vi "Arduino_Alterações_Labview.vi"() -> ()   [LabVIEW 2022 SP3]
uses:
  Program Files/National Instruments/LabVIEW 2022/examples/Instrument IO/Serial/support/Serial - XON-XOFF Characters.ctl
  Program Files/National Instruments/LabVIEW 2022/examples/Instrument IO/Serial/support/Serial - ASCII Characters.ctl
  Program Files/National Instruments/LabVIEW 2022/examples/Instrument IO/Serial/support/Serial - Settings.ctl
  <vilib>/Instr/_visa.llb/VISA Configure Serial Port (Instr).vi
  <vilib>/Utility/file.llb/Write Delimited Spreadsheet (DBL).vi
panel:
  out "Waveform Chart":dbl[][](graph)=[[24.999997972053873, 9.957040000000006, -52.0]]
  in  "dt (s)":dbl
  out "Water level (real) (m)":dbl
  in  "file (use dialog)":path
  in  "AI0_Ofset":dbl=50.0
  in  "AI0_Gain":dbl=-0.25 format="%#_13g"
  out "AI1":i32=511
  out "AI0":i32=418
  in  "VISA resource name":refnum<visa-resource-name>="COM4"
  in  "stop":bool
  # "Aquisition Parameters"
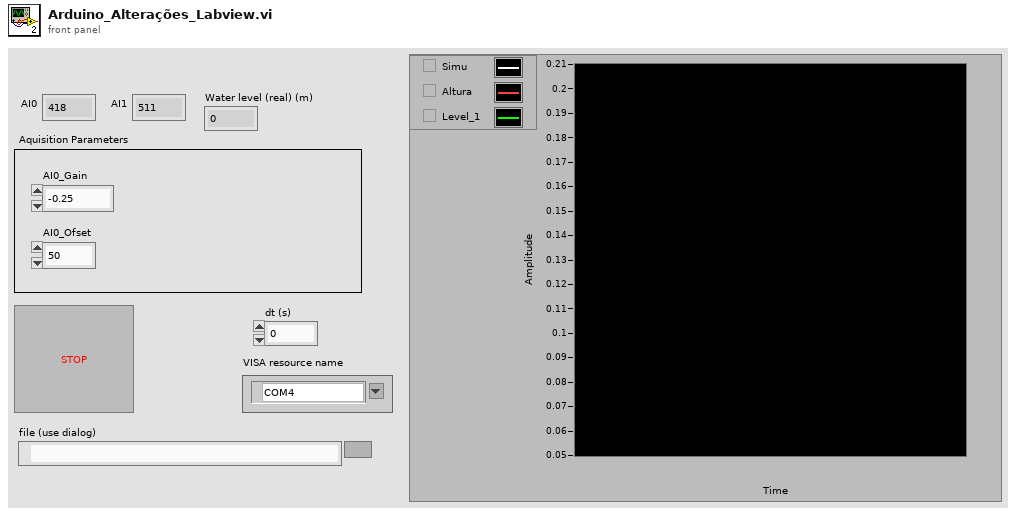
[diagram p1: front panel]
types:
  T1 = typedef "Serial - Settings.ctl" = cluster{"baud rate":u32, "data bits":u16, "parity":enum16{"None", "Odd", "Even", "Mark", "Space"}, "stop bits":u16, "flow control":u16}
  T2 = typedef "Serial - XON-XOFF Characters.ctl" = cluster{"XON":T3, "XOFF":T3}
  T3 = typedef "Serial - ASCII Characters.ctl" = enum16{"NUL", "SOH", "STX", "ETX", "EOT", "ENQ", "ACK", "BEL", "BS", "HT", "LF", "VT", "FF", "CR", "SO", "SI", "DLE", "DC1", "DC2", "DC3", "DC4", "NAK", "SYN", "ETB", "CAN", "EM", "SUB", "ESC", "FS", "GS", "RS", "US", "SP", "!", "\"", "#", "$", "%", "&", "'", "(", ")", "*", "+", ",", "- (-)", ".", "/", "0", "1", "2", "3", "4", "5", "6", "7", "8", "9", ":", ";", "<", "=", ">", "?", "@", "A", "B", "C", "D", "E", "F", "G", "H", "I", "J", "K", "L", "M", "N", "O", "P", "Q", "R", "S", "T", "U", "V", "W", "X", "Y", "Z", "[", "\\", "]", "^", "_", "`", "a", "b", "c", "d", "e", "f", "g", "h", "i", "j", "k", "l", "m", "n", "o", "p", "q", "r", "s", "t", "u", "v", "w", "x", "y", "z", "{", "|", "}", "~"}
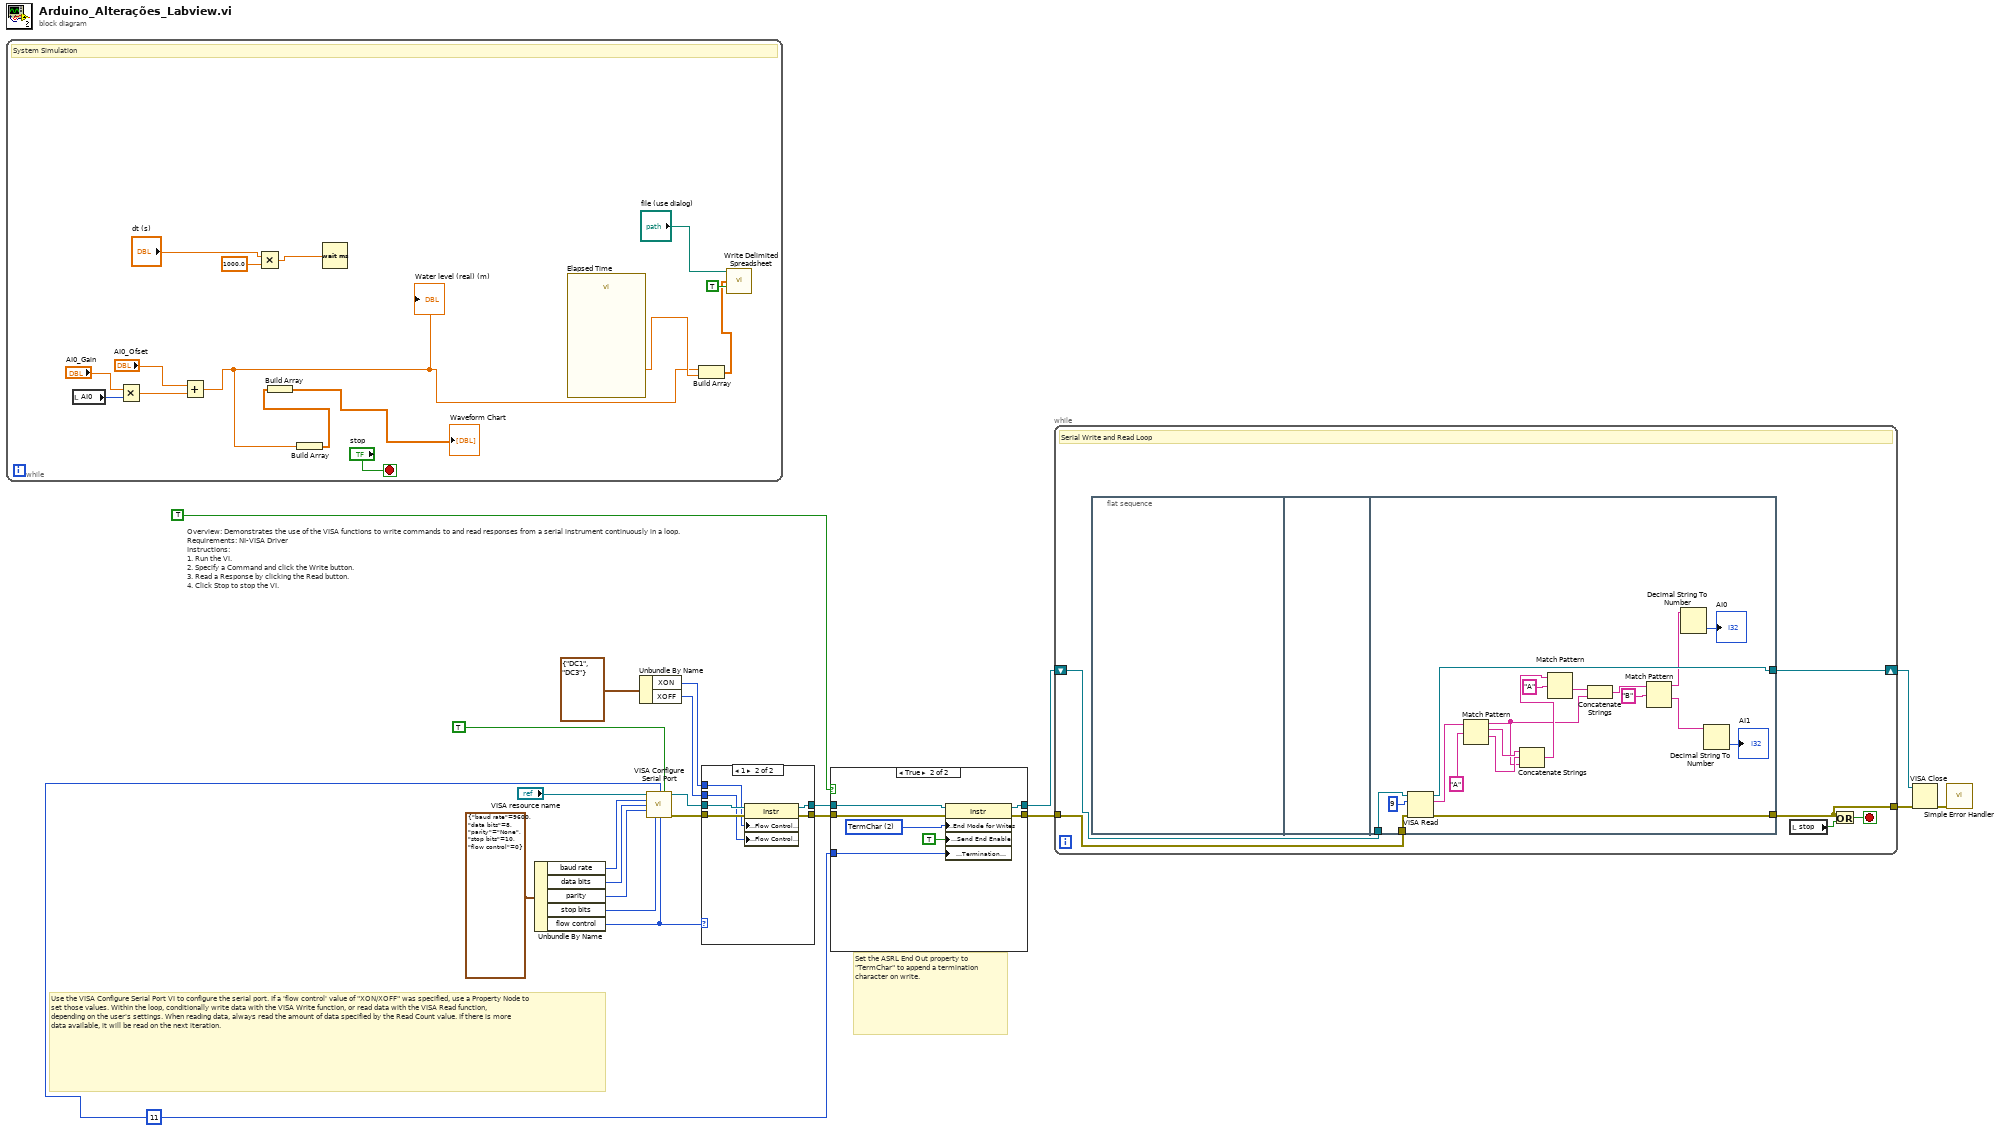
[diagram p0: block diagram]
diagram:
  w1 = u8 11 ("Termination Character")
  # "Set the ASRL End Out property to \"TermChar\" to append a termination character on write."
  # "Use the VISA Configure Serial Port VI to configure the serial port. If a 'flow control' value of \"XON/XOFF\" was specified, use a Property Node to set those values. Within the loop, conditionally write data with the VISA Write function, or read data with the VISA Read function, depending on the user's settings. When reading data, always read the amount of data specified by the Read Count value. If there is more data available, it will be read on the next iteration."
  # "Overview: Demonstrates the use of the VISA functions to write commands to and read responses from a serial instrument continuously in a loop.\nRequirements: NI-VISA Driver\nInstructions:\n1. Run the VI.\n2. Specify a Command and click the Write button.\n3. Read a Response by clicking the Read button.\n4. Click Stop to stop the VI."
  n1 = while {
    stop <- "stop" stop-if-true
    # "System Simulation"
    n2 = local read "AI0"() -> (w32:i32)
    n3 = Multiply(x="AI0_Gain", y=w32) -> (x*y=w35:dbl)
    n4 = Add(x="AI0_Ofset", y=w35) -> (x+y=w27:dbl)
    "Water level (real) (m)" <- w27
    n5 = Multiply(x="dt (s)", y=1000.0) -> (x*y=w25:dbl)
    n6 = Build Array(w27) -> (w33:dbl[])
    n7 = Build Array(w33) -> (→"Waveform Chart":dbl[][])
    n8 = Wait (ms)(milliseconds to wait=w25) -> ()  [unwired: 1 out]
    n9 = call "Elapsed Time"() -> ("Elapsed Time (s)"=w29:dbl)  [unwired: 12 in, 7 out]
    n10 = Build Array(w27, w29) -> (w28:dbl[])
    n11 = call-poly <vilib>:"Write Delimited Spreadsheet.vi"("file path (dialog if empty)"="file (use dialog)", "1D data"=w28, "append to file? (new file:F)"=TRUE) -> ()  [unwired: 11 in, 2 out]
  }
  n12 = Unbundle By Name(T1 {"baud rate"=9600, "data bits"=8, "parity"=enum."None", "stop bits"=10, "flow control"=0} ("Serial Settings")) -> ("baud rate"=w15:u32, "data bits"=w16:u16, "parity"=w17:enum16{"None", "Odd", "Even", "Mark", "Space"}, "stop bits"=w18:u16, "flow control"=w9:u16)
  n13 = Unbundle By Name(T2 {"XON"=enum."DC1", "XOFF"=enum."DC3"} ("XON/XOFF Characters")) -> ("XON"=w8:T3, "XOFF"=w7:T3)
  n14 = call-poly "VISA Configure Serial Port"("VISA resource name"="VISA resource name", "termination char\n(0xA = '\\n' = LF)"=w1, "Enable Termination\nChar (T)"=TRUE ("End Read on Termination Character?"), "baud rate (9600)"=w15, "data bits (8)"=w16, "parity (0:none)"=w17, "stop bits (10: 1 bit)"=w18, "flow control (0:none)"=w9) -> ("VISA resource name out"=w19:refnum<visa-resource-name>, "error out"=w20:errorcluster)  [unwired: 2 in, 4 out]
  n15 = case shown="1" w9 {
    tunnel: [w38 w45] -> w6
    tunnel: [w39 w44] -> w4
    tunnel: w20 -> [w38 w43]
    tunnel: w19 -> [w39 w42]
    tunnel: w8 -> [_ w41]
    tunnel: w7 -> [_ w40]
    frame Default {
    }
    frame 1 {
      n16 = property class="Instr"(reference=w42, error in=w43, "Serial Settings:Flow Control XON Character"=w41, "Serial Settings:Flow Control XOFF Character"=w40) -> (reference out=w44:refnum<visa-resource-name>, error out=w45:errorcluster)
    }
  }
  n17 = case shown="True" TRUE ("End Write on Termination Character?") {
    tunnel: w4 -> [w46 w54]
    tunnel: w6 -> [w47 w53]
    tunnel: [w46 w52] -> w3
    tunnel: [w47 w51] -> w5
    tunnel: w1 -> [_ w49]
    frame False {
    }
    frame True {
      w50 = u16 2 items=["None", "LastBit", "TermChar", "Break"] ("Serial Settings:Serial End Mode for Writes")
      n18 = property class="Instr"(reference=w54, error in=w53, "Serial Settings:End Mode for Writes"=w50, "Message Based Settings:Send End Enable"=TRUE, "Message Based Settings:Termination Character"=w49) -> (reference out=w52:refnum<visa-resource-name>, error out=w51:errorcluster)
    }
  }
  n19 = while {
    shift-right: [w60] -> w10
    shift-left: w3 -> [w55]
    tunnel: w5 -> [w56]
    tunnel: [w58] -> w11
    stop <- w59 stop-if-true
    # "Serial Write and Read Loop"
    n20 = flat-sequence {
      tunnel: [w79] -> w60
      tunnel: [w78] -> w58
      tunnel: w56 -> [w62]
      tunnel: w55 -> [w61]
      frame #0 {
      }
      frame #1 {
      }
      frame #2 {
        n21 = VISA Read(VISA resource name=w61, byte count=u32 9 ("Read Count"), error in (no error)=w62) -> (VISA resource name out=w79:refnum<visa-resource-name>, read buffer=w63:string, error out=w78:errorcluster)  [unwired: 1 out]
        n22 = Match Pattern(string=w63, regular expression="A") -> (before substring=w66:string, match substring=w68:string, after substring=w67:string)  [unwired: 1 in, 1 out]
        n23 = Concatenate Strings(w68, w67, w66) -> (w69:string)
        n24 = Match Pattern(string=w69, regular expression="A") -> (after substring=w72:string)  [unwired: 1 in, 3 out]
        n25 = Concatenate Strings(w72, w66) -> (w71:string)
        n26 = Match Pattern(string=w71, regular expression="B") -> (before substring=w65:string, after substring=w64:string)  [unwired: 1 in, 2 out]
        n27 = Decimal String To Number(string=w65) -> (number=→"AI0":i32)  [unwired: 2 in, 1 out]
        n28 = Decimal String To Number(string=w64) -> (number=→"AI1":i32)  [unwired: 2 in, 1 out]
      }
    }
    n29 = local read "stop"() -> (w57:bool)
    n30 = Or(x=w58, y=w57) -> (x .or. y?=w59:bool)
  }
  n31 = VISA Close(VISA resource name=w10, error in (no error)=w11) -> (error out=w12:errorcluster)
  n32 = call <vilib>:"Simple Error Handler.vi"("error in (no error)"=w12) -> ()  [unwired: 1 in, 8 out]
